vi "writeReadPistofono.vi"(8 "error in (no error)":errorcluster, 10 "Command":string="*IDN?", 11 "Pistofono in":refnum<class "Pistofono.lvclass">) -> (0 "error out":errorcluster, 2 "medicion (num)":dbl, 3 "Pistofono out":refnum<class "Pistofono.lvclass">)   [LabVIEW 2019, in "Pistofono.lvclass"]
uses:
  Pistofono.lvclass
  Pistofono.lvclass/Pistofono.ctl
panel:
  out "medicion":string
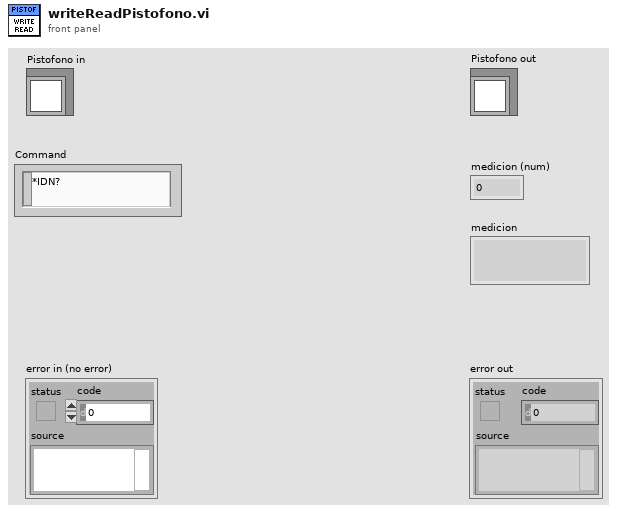
[diagram p1: front panel]
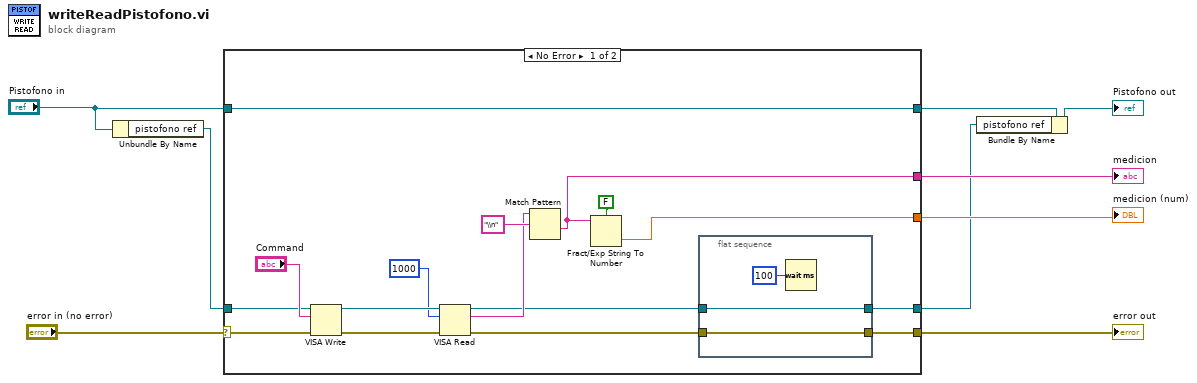
[diagram p0: block diagram]
diagram:
  n1 = Unbundle By Name("Pistofono in") -> ("pistofono ref"=w3:refnum<visa-resource-name>)
  n2 = case shown="No Error" "error in (no error)" {
    selector: "error in (no error)" -> [w20 w31]
    tunnel: [w11 w31] -> w8
    tunnel: [w25 w30] -> w7
    tunnel: "Pistofono in" -> [w25 w30]
    tunnel: [w13 w29] -> w1
    tunnel: [w16 _] -> w6
    tunnel: [w15 _] -> w5
    tunnel: w3 -> [w14 w29]
    frame No Error {
      n3 = VISA Write(VISA resource name=w14, write buffer="Command", error in (no error)=w20) -> (VISA resource name out=w24:refnum<visa-resource-name>, error out=w23:errorcluster)  [unwired: 1 out]
      n4 = VISA Read(VISA resource name=w24, byte count=u32 1000 ("Read Count"), error in (no error)=w23) -> (VISA resource name out=w12:refnum<visa-resource-name>, read buffer=w18:string, error out=w10:errorcluster)  [unwired: 1 out]
      n5 = Match Pattern(string=w18, regular expression="\\n") -> (after substring=w15:string)  [unwired: 1 in, 3 out]
      n6 = Fract/Exp String To Number(use system decimal point (T)=FALSE, string=w15) -> (number=w16:dbl)  [unwired: 2 in, 1 out]
      n7 = flat-sequence {
        tunnel: [w28] -> w13
        tunnel: w12 -> [w28]
        tunnel: [w27] -> w11
        tunnel: w10 -> [w27]
        frame #0 {
          n8 = Wait (ms)(milliseconds to wait=u32 100) -> ()  [unwired: 1 out]
        }
      }
    }
    frame Error {
    }
  }
  "error out" <- w8
  "medicion" <- w5
  "medicion (num)" <- w6
  n9 = Bundle By Name(cluster=w7, "pistofono ref"=w1) -> (→"Pistofono out":refnum<class "Pistofono.lvclass">)
